vi "X Listbox Update for Add and Delete.vi"(10 "Names":string[](array[string]), 11 "# Items":i32) -> (1 "Item Symbols":i32[](array[numeric]), 2 "Active Row":i32, 3 "Name":string)   [LabVIEW 2011, in "X Listbox-Solution.xctl"]
doc: "This subVI is used in the creation of the facade for the X Listbox XControl.\n\nAAL 9/09"
uses:
  X Listbox-Solution.xctl
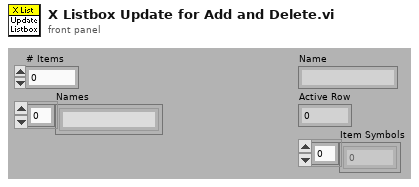
[diagram p1: front panel]
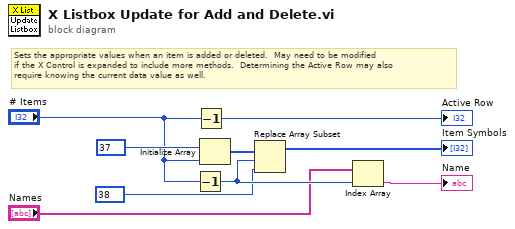
[diagram p0: block diagram]
diagram:
  # "Sets the appropriate values when an item is added or deleted.  May need to be modified \nif the X Control is expanded to include more methods.  Determining the Active Row may also\nrequire knowing the current data value as well."
  n1 = Decrement(x="# Items") -> (x-1=w6:i32)
  n2 = Decrement(x="# Items") -> (x-1=→"Active Row":i32)
  n3 = Initialize Array(37, "# Items") -> (w2:i32[])
  n4 = Replace Array Subset(array=w2, new element=38, index=w6) -> (→"Item Symbols":i32[])
  n5 = Index Array(array="Names", index=w6) -> (element=→"Name":string)
